vi "Test_NestedLog_StartStop_ParentNotStopped.vi"(8 "error in (no error)":errorcluster, 11 "TestCase in":refnum<class "TestAggregateLog.lvclass">) -> (0 "error out":errorcluster, 3 "TestCase out":refnum<class "TestAggregateLog.lvclass">)   [LabVIEW 2017, in "TestAggregateLog.lvclass"]
uses:
  TestAggregateLog.lvclass
  Source/LVQueue Sink/LVQueue Sink.lvclass/LVQueue Sink.ctl
  Source/Composed Log/LoggerReference/LoggerReference.lvclass/LoggerReference.ctl
  007c25be-df45-44e6-bcd0-86f151692ed8.vi
  0b3f8f0b-b660-41ef-a979-373f01dd03ae.vi
  Source/Composed Log/LoggerReference/Return Aggregate Queues.vi
  Source/Composed Log/LoggerReference/Add Aggregate Log.vi
  007c25be-df45-44e6-bcd0-86f151692ed8.vi/fa4e5d10-78c6-4c84-881b-f1e8d498449c.vi
  0b3f8f0b-b660-41ef-a979-373f01dd03ae.vi/1348330f-7379-436e-a353-a00fd891c483.vi
  Source/Composed Log/LoggerReference/Log.vi
  Source/Composed Log/LoggerReference/Get Valid Event Time.vi
  Source/Composed Log/LoggerReference/Send Add Sink.vi
  Source/Composed Log/LoggerReference/Remove Stale Logs.vi
  Source/LVQueue Sink/LVQueue Sink.lvclass
  C:/CS/Internal/LabVIEW/Logger/Source/Composed Log/Log Sink/Log Sink.lvclass
  Source/Composed Log/Application Logger/Launch Worker Loop.vi
  Source/Composed Log/LoggerReference/Initialize Logger Instance.vi
  Source/Composed Log/LoggerReference/LoggerReference.lvclass
  Source/Composed Log/IErrorFormat/IErrorFormat.lvclass
  Source/Composed Log/Log Sink/Log Sink.lvclass
  <vilib>/addons/_JKI Toolkits/VI Tester/TestCase.llb/TestCase.lvclass
  C:/Program Files (x86)/National Instruments/LabVIEW 2017/vi.lib/addons/_JKI Toolkits/VI Tester/TestCase.llb/TestCase.lvclass
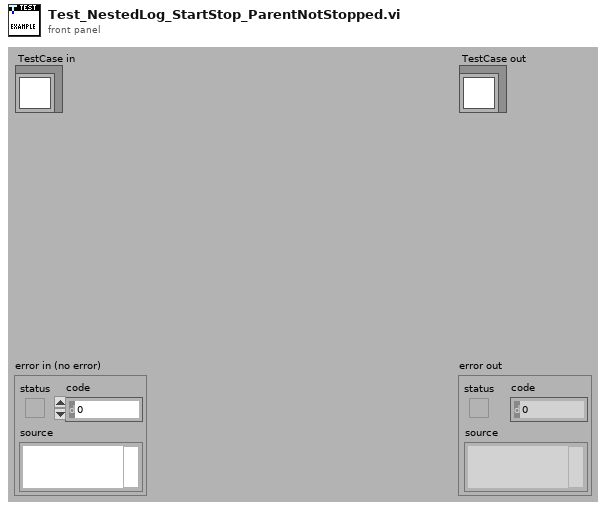
[diagram p1: front panel]
types:
  T1 = typedef "Composed Log.lvlib/Log Packet.ctl" = cluster{"Data To Log":string, "Source":string, "Event Level":T2, "Event Time":timestamp}
  T2 = typedef "Composed Log.lvlib/Log Level.ctl" = enum16{"Debug", "Info", "Warning", "Error", "Critical"}
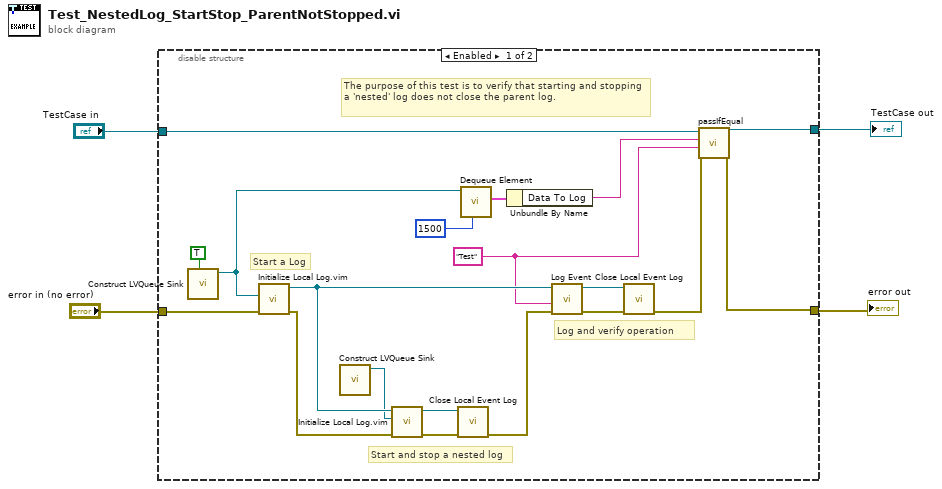
[diagram p0: block diagram]
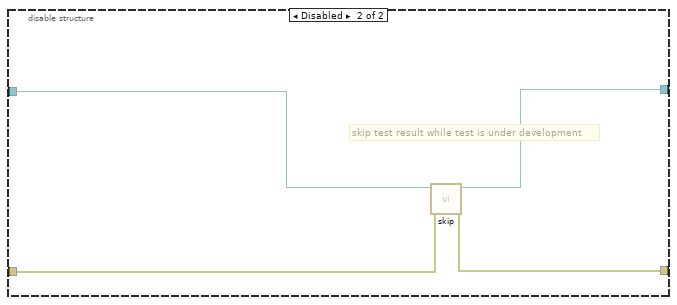
[diagram p2: hidden frame]
diagram:
  n1 = disable-structure "This diagram is for convenience to enable skipping a test easily (enable 'Skip' case)" shown="Enabled" {
    disable-tunnel: "TestCase in" -> [w23 w27]
    disable-tunnel: [w22 w25] -> w1
    disable-tunnel: [w21 w26] -> w3
    disable-tunnel: "error in (no error)" -> [w20 w24]
    frame Enabled {
      w7 = "Test" ("SourceID")
      # "The purpose of this test is to verify that starting and stopping a 'nested' log does not close the parent log."
      # "Log and verify operation"
      # "Start and stop a nested log"
      # "Start a Log"
      n2 = call "Construct LVQueue Sink.vi"("User Shutdown? (F)"=TRUE) -> ("LVQueue Sink out"=w6:refnum<class "LVQueue Sink.lvclass">)  [unwired: 9 in, 1 out]
      n3 = call "Initialize Local Log.vim"("error in (no error)"=w20, "Startup Sink(s)"=w6) -> ("error out"=w19:errorcluster, "Log Instance Reference"=w10:refnum<class "LoggerReference.lvclass">)  [unwired: 7 in, 1 out]
      n4 = call "Construct LVQueue Sink.vi"() -> ("LVQueue Sink out"=w5:refnum<class "LVQueue Sink.lvclass">)  [unwired: 10 in, 1 out]
      n5 = call "Initialize Local Log.vim"("error in (no error)"=w19, "Startup Sink(s)"=w5, "Parent Log Reference"=w10) -> ("error out"=w16:errorcluster, "Log Instance Reference"=w17:refnum<class "LoggerReference.lvclass">)  [unwired: 6 in, 1 out]
      n6 = call "Close Local Event Log.vi"("error in (no error)"=w16, "Log Instance"=w17) -> ("error out"=w18:errorcluster)  [unwired: 9 in]
      n7 = call "Dequeue Element.vi"("timeout in ms (-1)"=1500, "LVQueue Sink in"=w6) -> ("Log Packet"=w9:T1)  [unwired: 6 in, 3 out]
      n8 = Unbundle By Name(w9) -> ("Data To Log"=w8:string)
      n9 = call "Log Event.vi"("error in (no error)"=w18, "Data To Log"=w7, "Log Instance"=w10) -> ("error out"=w13:errorcluster, "Log Instance Out"=w12:refnum<class "LoggerReference.lvclass">)  [unwired: 7 in]
      n10 = call "Close Local Event Log.vi"("error in (no error)"=w13, "Log Instance"=w12) -> ("error out"=w11:errorcluster)  [unwired: 9 in]
      n11 = call-dynamic "passIfEqual.vi"("error in (no error)"=w11, "y"=w7, "x"=w8, "TestCase in"=w23) -> ("error out"=w21:errorcluster, "TestCase out"=w22:refnum<class "TestAggregateLog.lvclass">)  [unwired: 6 in]
    }
    frame Disabled {
      # "skip test result while test is under development"
      n12 = call <vilib>:"skip.vi"("error in (no error)"=w24, "TestCase in"=w27) -> ("error out"=w26:errorcluster, "TestCase out"=w25:refnum<class "TestAggregateLog.lvclass">)  [unwired: 8 in]
    }
  }
  "error out" <- w3
  "TestCase out" <- w1
